vi "FT_Get_Device_Description_By_Index.vi"(0 "Device Index":u32, 11 "Error In":errorcluster) -> (4 "FT_Status":u32(ring) items=["FT_OK", "FT_INVALID_HANDLE", "FT_DEVICE_NOT_FOUND", "FT_DEVICE_NOT_OPENED", "FT_IO_ERROR", "FT_INSUFFICIENT_RESOURCES", "FT_INVALID_PARAMETER", "FT_INVALID_BAUD_RATE", "FT_DEVICE_NOT_OPENED_FOR_ERASE", "FT_DEVICE_NOT_OPENED_FOR_WRITE", "FT_FAILED_TO_WRITE_DEVICE", "FT_EEPROM_READ_FAILED", "FT_EEPROM_WRITE_FAILED", "FT_EEPROM_ERASE_FAILED", "FT_EEPROM_NOT_PRESENT", "FT_EEPROM_NOT_PROGRAMMED", "FT_INVALID_ARGS", "FT_NOT_SUPPORTED", "FT_OTHER_ERROR"], 6 "Device Description":string, 15 "Error Out":errorcluster)   [LabVIEW 2020]
uses:
  GEA3 DLL Source/ftd2xx.dll
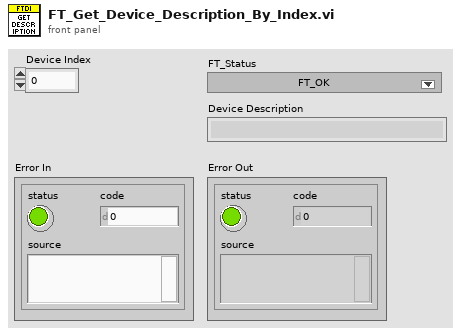
[diagram p1: front panel]
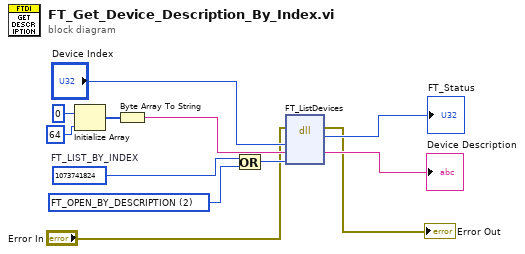
[diagram p0: block diagram]
diagram:
  w9 = u32 2 items=["FT_OPEN_BY_SERIAL_NUMBER"=1, "FT_OPEN_BY_DESCRIPTION"=2, "FT_OPEN_BY_LOCATION"=4] ("Flags")
  w8 = u32 1073741824  # FT_LIST_BY_INDEX
  n1 = Initialize Array(u8 0, 64 ("dimension size")) -> (w5:u8[])
  n2 = Byte Array To String(unsigned byte array=w5) -> (string=w4:string)
  n3 = Or(x=w8, y=w9) -> (x .or. y?=w7:u32)
  n4 = dll-call lib="C:/TechnologyLab/NI-2010/Drivers/GEA3 Toolkit/GEA3 DLL Source/ftd2xx.dll" fn="FT_ListDevices"(error in="Error In", "DeviceIndex"="Device Index", "DeviceDescription"=w4, "Flags"=w7) -> (error out=→"Error Out":errorcluster, "FT_Status"=→"FT_Status":u32, "DeviceDescription"=→"Device Description":string)  [unwired: 4 in, 1 out]
